vi "sys_front_panel_V1.vi"() -> ()   [LabVIEW 2024]
uses:
  <vilib>/Analysis/1siggen.llb/Ramp Pattern by Samples.vi
  <vilib>/Analysis/NI_AALBase.lvlib
panel:
  out "WRx 2 Spectrum Plot":cluster{"Y":dbl[], "Y":dbl[]}[](graph)
  in  "RTHost Selection":u16(ring) items=["192.168.1.2 C011T D83198", "192.168.1.4 C011T 50E219"]
  in  "Scan for\nConfig":bool
  out "Hardware\nBusy":bool
  in  "Toggle\nMeasurement":bool
  in  "Spectrum Sampling Period (s)":dbl caption="Measured\nOperating \nFrequency" format="%#_4f"
  out "WRx 1 Spectrum Plot":cluster{"Y":dbl[], "Y":dbl[]}[](graph)
  in  "FlexCompute Selection":u16(ring) items=["192.168.1.1 C100T 909B13", "192.168.1.3 C100T 4363DA"]
  in  "FlexSDR Selection":u16(ring) items=["192.168.1.5  S8010-01 9770BC", "192.168.1.6  S8010-01 24BD53"]
  in  "Stop Program":bool
  in  "Use Random\nDevices":bool
  in  "Scan for \nDevices":bool
  in  "?":T1(tab)
  in  "Runtime\nCalibration":bool
  in  "?":enum32{"WRx 1", "WRx 2"}(tab)
  in  "WRx 1\nGain Attenuation":i64(knob) caption="RX Gain Attenuation" min=0 max=27 step=1 scale=0.0..27.0
  in  "WRx 1\nIF Frequency":u16(ring) caption="IF Frequency" items=["1200 MHz", "1400 MHz", "3000 MHZ"]
  in  "WRx 1\nEnable Channel":bool caption="Enable \nChannel"
  in  "WRx 1\nBandwidth Mode":u16(ring) caption="Bandwidth Mode" items=["500 MHz"]
  in  "WRx 1\nGain Mode":u16(ring) caption="Gain Mode" items=["Automatic", "Fixed"]
  in  "WRx 1\nRSSI Threshold":dbl caption="RX RSSI Threshold" format="%.2f dBm"
  in  "WRx 2\nGain Mode":u16(ring) caption="Gain Mode" items=["Automatic", "Fixed"]
  in  "WRx 2\nBandwidth Mode":u16(ring) caption="Bandwidth Mode" items=["500 MHz"]
  in  "WRx 2\nEnable Channel":bool caption="Enable \nChannel"
  in  "WRx 2\nIF Frequency":u16(ring) caption="IF Frequency" items=["1200 MHz", "1400 MHz", "3000 MHZ"]
  in  "WRx 2\nGain Attenuation":i64(knob) caption="RX Gain Attenuation" min=0 max=27 step=1 scale=0.0..27.0
  in  "WRx 2\nRSSI Threshold":dbl caption="RX RSSI Threshold" format="%.2f dBm"
  in  "Update \nConfiguration":bool
  in  "Doppler\nBypass":bool
  in  "Pre-Trigger Time":dbl format="%.3f ms"
  in  "Post-Trigger Time":dbl format="%.3f ms"
  in  "Trigger Type":u16(ring) items=["GPS Time", "Anomaly Detection"]
  in  "Trigger Frequency":u16(ring) caption="Trigger Type" items=["Single", "Continuous"]
  out "WRx 2 \nGain Attenuation":dbl caption="WRx 2 Gain Attenuation" format="%.0f dBm"
  out "WRx 1 \nGain Attenuation":dbl caption="WRx 1 Gain Attenuation" format="%.0f dBm"
  in  "WRx Scan":bool
  out "WRx 1 RSSI":dbl caption="Measured\nOperating \nFrequency" format="%.2f dBm"
  in  "HW Reset":bool
  in  "Self-Cal":bool
  out "WRx 2 RSSI":dbl caption="Measured\nOperating \nFrequency" format="%.2f dBm"
  out "WRx 2 En":bool
  out "WRx 1 En":bool
  out "RTHost\nDevices":string[][](array[string])
  out "FlexCompute\nDevices":string[][](array[string])
  out "FlexSDR\nDevices":string[][](array[string])
  out "Measurement\nActive":bool
  out "GPS \nLOCK":bool
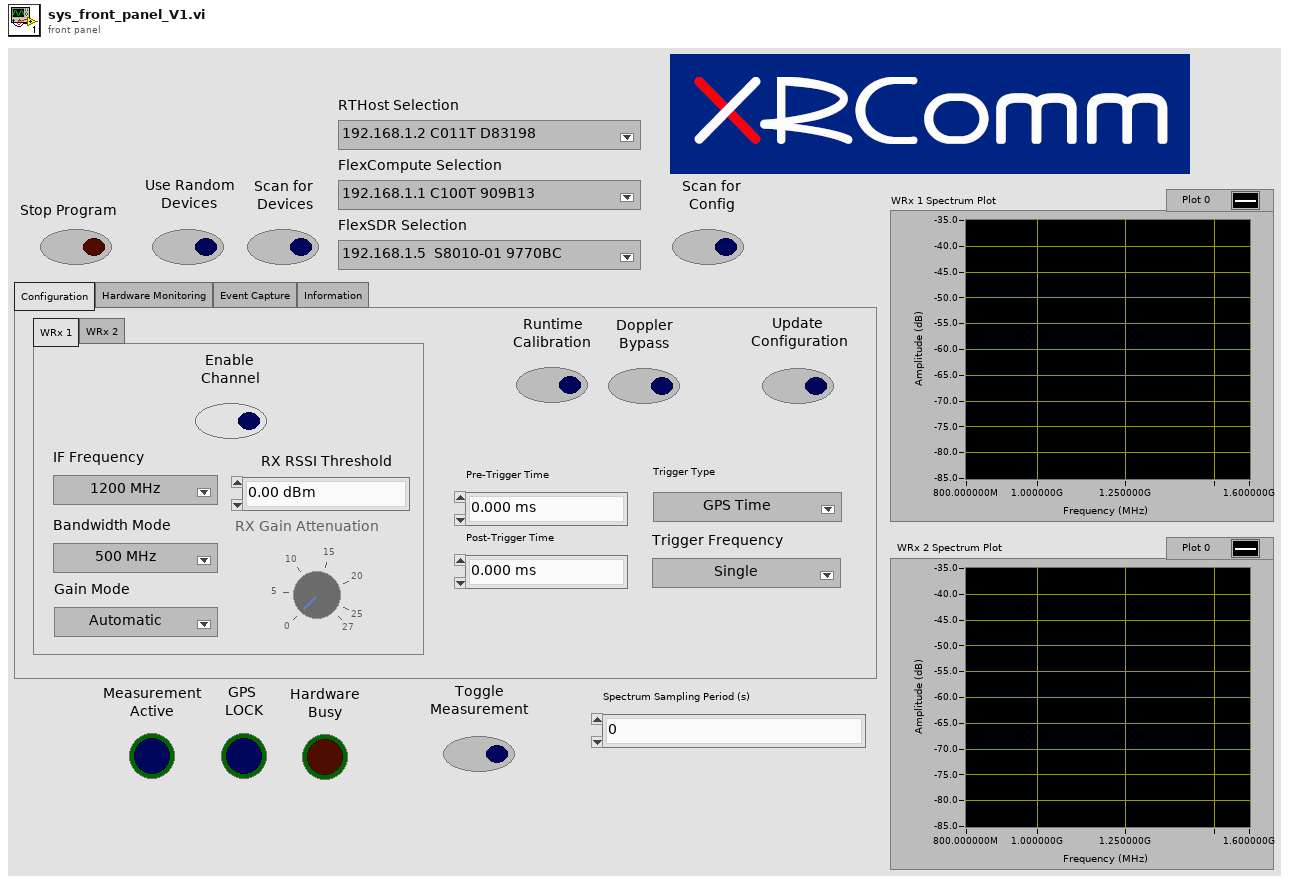
[diagram p1: front panel]
types:
  T1 = enum32{"Configuration", "Hardware Monitoring", "Event Capture", "Information"}
  T2 = enum8{"Enabled", "Disabled", "Disabled and Grayed Out"}
  T3 = cluster{"RTHost Selection":u16, "FlexCompute Selection":u16, "FlexSDR Selection":u16}
  T4 = cluster{"RTHost\nDevices":string[][], "FlexCompute\nDevices":string[][], "FlexSDR\nDevices":string[][]}
  T5 = cluster{"Doppler\nBypass":bool, "Trigger Type":u16, "Trigger Frequency":u16, "Pre-Trigger Time":dbl, "Post-Trigger Time":dbl}
  T6 = cluster{"WRx 1\nEnable Channel":bool, "WRx 1\nIF Frequency":u16, "WRx 1\nBandwidth Mode":u16, "WRx 1\nGain Mode":u16, "WRx 1\nRSSI Threshold":dbl, "WRx 1\nGain Attenuation":i64, "WRx 2\nEnable Channel":bool, "WRx 2\nIF Frequency":u16, "WRx 2\nBandwidth Mode":u16, "WRx 2\nGain Mode":u16, "WRx 2\nRSSI Threshold":dbl, "WRx 2\nGain Attenuation":i64, "Runtime\nCalibration":bool, "Measurement\nActive":bool}
  T7 = cluster{"SDR Config":cluster{"WRx 1\nEnable Channel":bool, "WRx 1\nIF Frequency":u16, "WRx 1\nBandwidth Mode":u16, "WRx 1\nGain Mode":u16, "WRx 1\nRSSI Threshold":dbl, "WRx 1\nGain Attenuation":i64, "WRx 2\nEnable Channel":bool, "WRx 2\nIF Frequency":u16, "WRx 2\nBandwidth Mode":u16, "WRx 2\nGain Mode":u16, "WRx 2\nRSSI Threshold":dbl, "WRx 2\nGain Attenuation":i64, "Runtime\nCalibration":bool, "Measurement\nActive":bool}, "Compute Config":cluster{"Doppler\nBypass":bool, "Trigger Type":u16, "Trigger Frequency":u16, "Pre-Trigger Time":dbl, "Post-Trigger Time":dbl}}
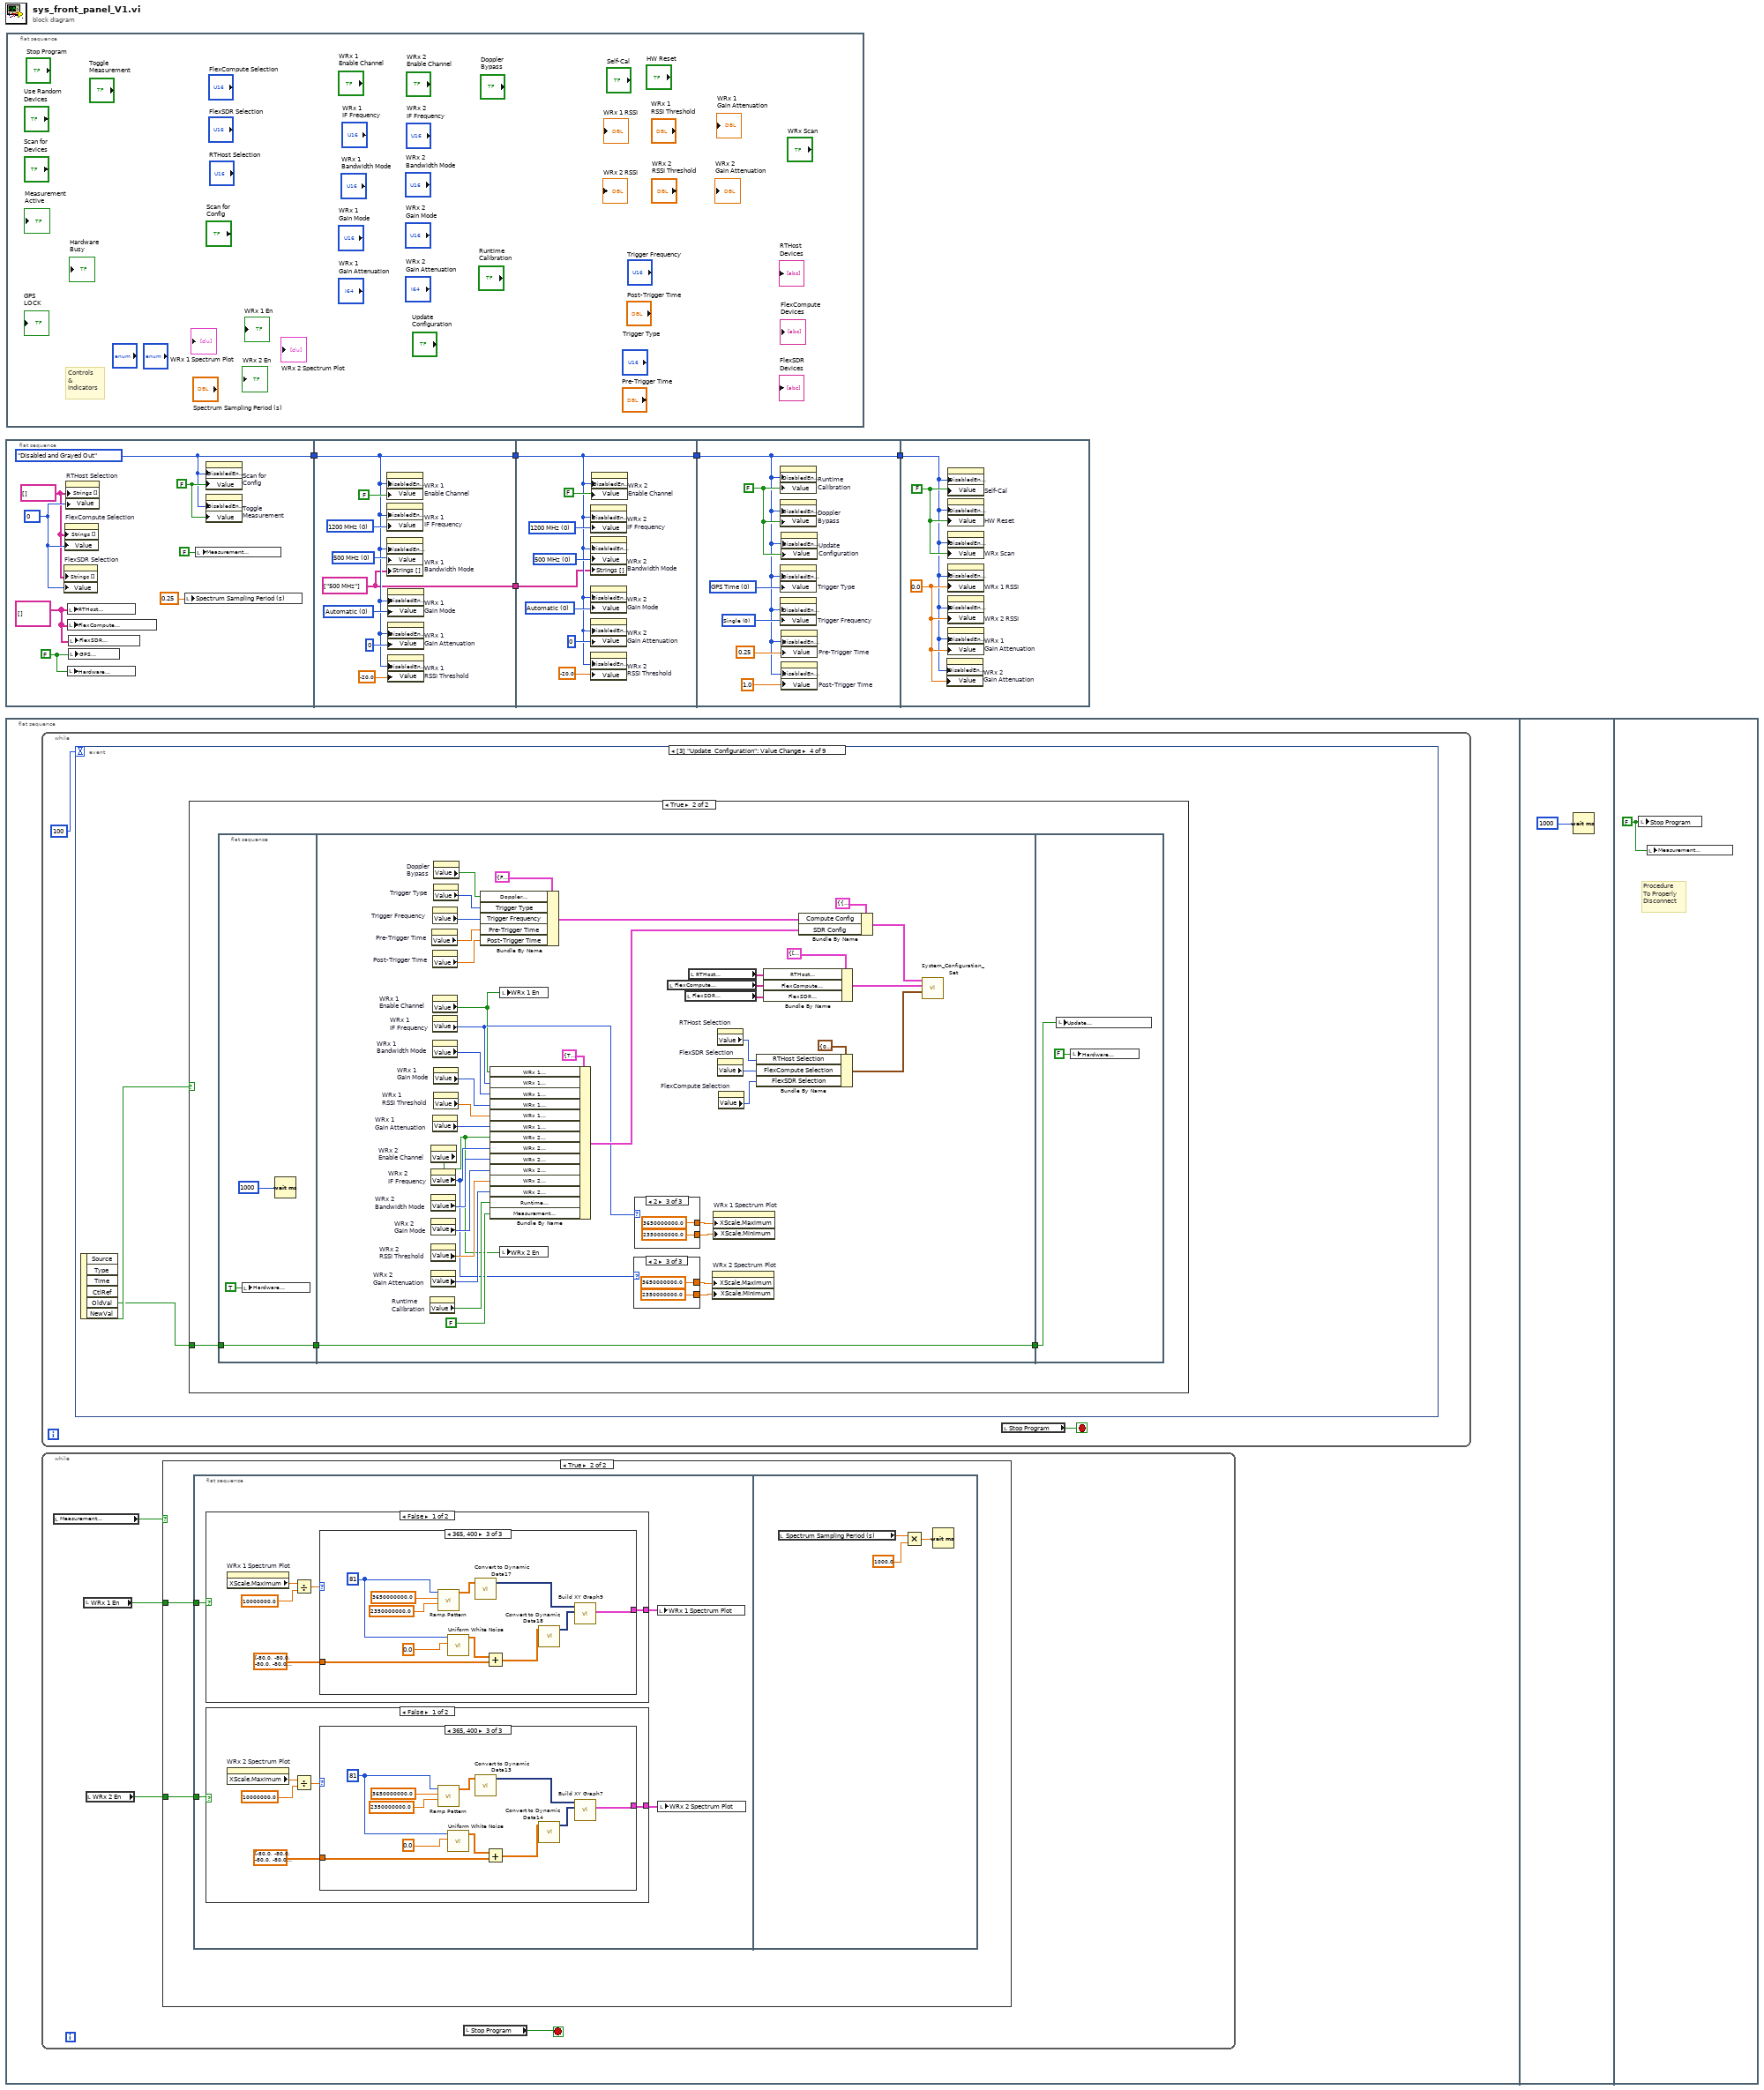
[diagram p0: block diagram]
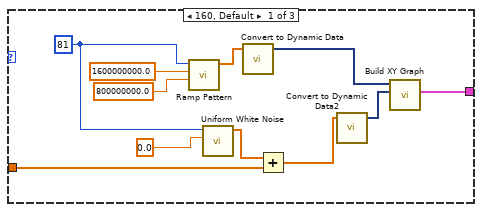
[diagram p3: hidden frame]
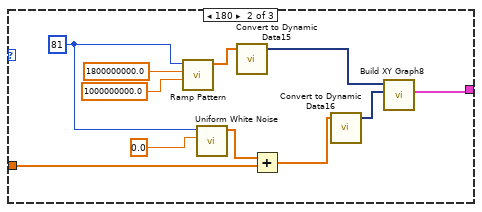
[diagram p4: hidden frame]
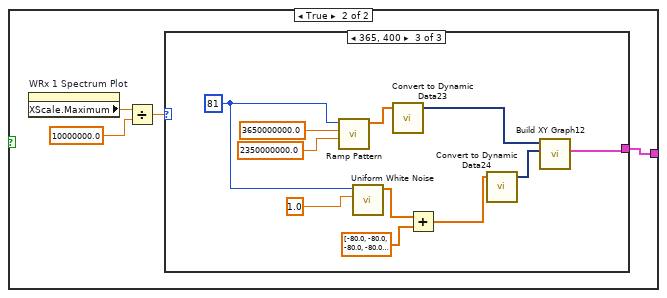
[diagram p5: hidden frame]
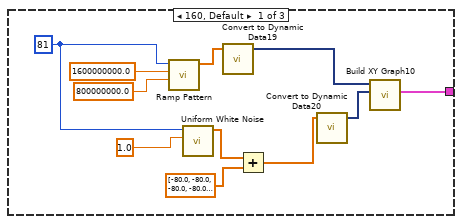
[diagram p6: hidden frame]
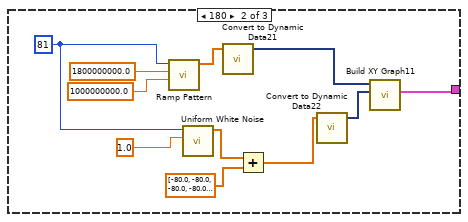
[diagram p7: hidden frame]
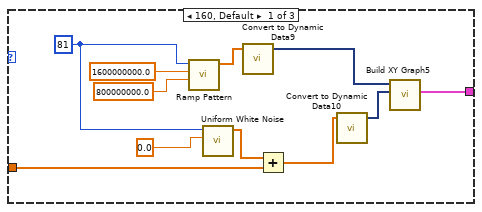
[diagram p8: hidden frame]
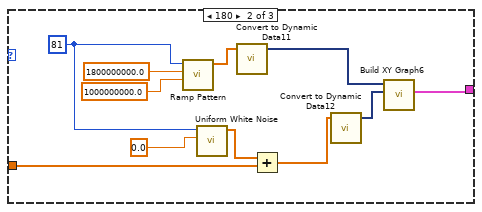
[diagram p9: hidden frame]
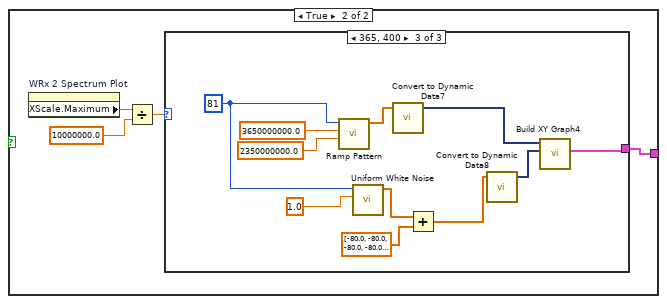
[diagram p10: hidden frame]
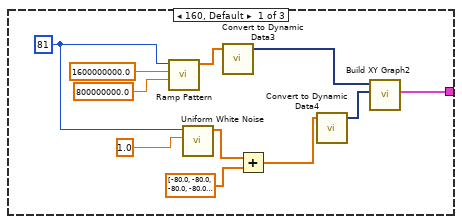
[diagram p11: hidden frame]
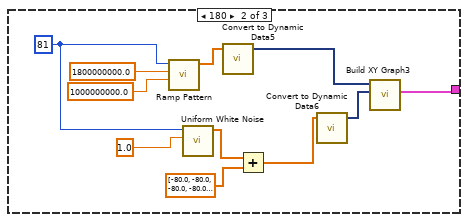
[diagram p12: hidden frame]
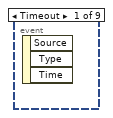
[diagram p13: hidden frame]
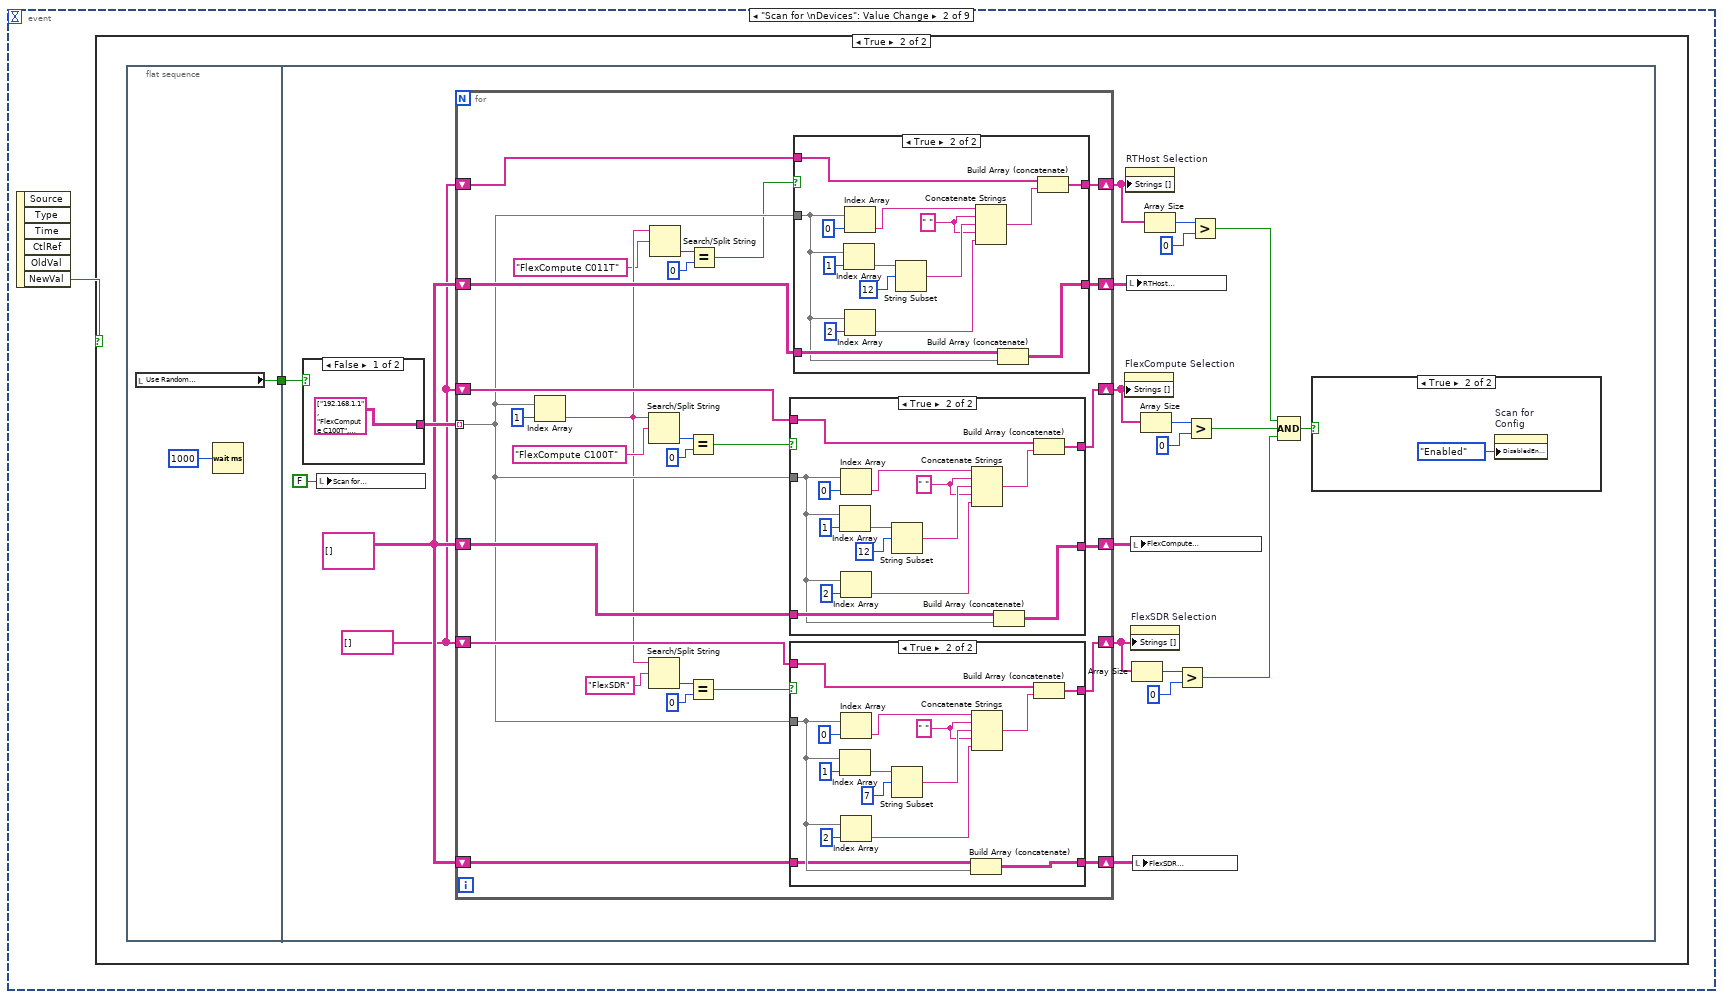
[diagram p14: hidden frame]
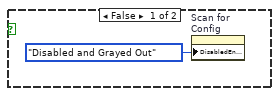
[diagram p16: hidden frame]
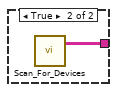
[diagram p20: hidden frame]
diagram:
  n1 = flat-sequence {
    frame #0 {
      n2 = while {
        stop <- w170 stop-if-true
        n3 = event shown="[3] \"Update  Configuration\": Value Change" {
          selector: _ -> [_ _ _ _ _ _ _ _ _]
          dyn-events: _ -> [_ _ _ _ _ _ _ _ _]
          timeout: 100 -> [_ _ _ _ _ _ _ _ _]
          event Timeout {
            n4 = event-data() -> ()  [unwired: 1 in, 3 out]
          }
          event "Scan for \nDevices": Value Change {
            n5 = event-data() -> ("NewVal"=w171:bool)  [unwired: 1 in, 5 out]
            n6 = case shown="True" w171 {
              frame False {
              }
              frame True {
                n7 = flat-sequence {
                  tunnel: [w173] -> w172
                  tunnel: w172 -> [w191]
                  frame #0 {
                    n8 = local read "Use Random\nDevices"() -> (w173:bool)
                    n9 = Wait (ms)(milliseconds to wait=u32 1000) -> ()  [unwired: 1 out]
                  }
                  frame #1 {
                    w190 = string[][] [] ("Flex Computer\nDevices 2")
                    w189 = string[] []
                    n10 = case shown="False" w191 {
                      tunnel: [string[][] [["192.168.1.1", "FlexCompute C100T", "909B13"], ["192.168.1.2", "FlexCompute C011T", "D83198"], ["192.168.1.3", "FlexCompute C100T", "4363DA"], ["192.168.1.4", "FlexCompute C011T", "50E219"], ["192.168.1.5", "FlexSDR S8010-01", "9770BC"], ["192.168.1.6", "FlexSDR S8010-01", "24BD53"]] ("Device Properties") w277] -> w194
                      frame False {
                      }
                      frame True {
                        n11 = call "Scan_For_Devices.vi"() -> ("Device Properties"=w277:string[][])  [unwired: 3 in]
                      }
                    }
                    n12 = local write "Scan for \nDevices"(FALSE ("Scan for \nDevices")) -> ()
                    n13 = for {
                      tunnel: w194 -> [w201] mode=indexing
                      shift-right: [w219] -> w182
                      shift-left: w189 -> [w220]
                      shift-right: [w218] -> w179
                      shift-left: w189 -> [w213]
                      shift-right: [w211] -> w193
                      shift-left: w190 -> [w212]
                      shift-right: [w209] -> w192
                      shift-left: w190 -> [w210]
                      shift-right: [w206] -> w188
                      shift-left: w190 -> [w207]
                      shift-right: [w205] -> w187
                      shift-left: w189 -> [w204]
                      n14 = Index Array(array=w201, index=1) -> (element=w200:string)
                      n15 = Search/Split String(string=w200, search string/char (-)="FlexCompute C100T") -> (offset of match=w223:i32)  [unwired: 1 in, 2 out]
                      n16 = Search/Split String(string=w200, search string/char (-)="FlexSDR") -> (offset of match=w217:i32)  [unwired: 1 in, 2 out]
                      n17 = Search/Split String(string=w200, search string/char (-)="FlexCompute C011T") -> (offset of match=w203:i32)  [unwired: 1 in, 2 out]
                      n18 = Equal?(x=w223, y=0) -> (x = y?=w221:bool)
                      n19 = Equal?(x=w217, y=0) -> (x = y?=w214:bool)
                      n20 = Equal?(x=w203, y=0) -> (x = y?=w198:bool)
                      n21 = case shown="True" w221 {
                        tunnel: w201 -> [_ w262]
                        tunnel: w220 -> [w260 w265]
                        tunnel: [w260 w264] -> w219
                        tunnel: w212 -> [w259 w263]
                        tunnel: [w259 w261] -> w211
                        frame False {
                        }
                        frame True {
                          w268 = " " ("string")
                          n22 = Index Array(array=w262, index=1) -> (element=w272:string)
                          n23 = Index Array(array=w262, index=0) -> (element=w270:string)
                          n24 = Index Array(array=w262, index=2) -> (element=w267:string)
                          n25 = String Subset(string=w272, offset (0)=12) -> (substring=w269:string)  [unwired: 1 in]
                          n26 = Concatenate Strings(w270, w268, w269, w268, w267) -> (w266:string)
                          n27 = Build Array (concatenate)(w263, w262) -> (w261:string[][])
                          n28 = Build Array (concatenate)(w265, w266) -> (w264:string[])
                        }
                      }
                      n29 = case shown="True" w214 {
                        tunnel: w201 -> [_ w246]
                        tunnel: w213 -> [w243 w248]
                        tunnel: [w243 w247] -> w218
                        tunnel: w210 -> [w242 w245]
                        tunnel: [w242 w244] -> w209
                        frame False {
                        }
                        frame True {
                          w251 = " " ("string")
                          n30 = Index Array(array=w246, index=1) -> (element=w255:string)
                          n31 = Index Array(array=w246, index=0) -> (element=w253:string)
                          n32 = Index Array(array=w246, index=2) -> (element=w250:string)
                          n33 = String Subset(string=w255, offset (0)=7) -> (substring=w252:string)  [unwired: 1 in]
                          n34 = Build Array (concatenate)(w245, w246) -> (w244:string[][])
                          n35 = Concatenate Strings(w253, w251, w252, w251, w250) -> (w249:string)
                          n36 = Build Array (concatenate)(w248, w249) -> (w247:string[])
                        }
                      }
                      n37 = case shown="True" w198 {
                        tunnel: w201 -> [_ w228]
                        tunnel: w204 -> [w226 w231]
                        tunnel: [w226 w230] -> w205
                        tunnel: w207 -> [w225 w229]
                        tunnel: [w225 w227] -> w206
                        frame False {
                        }
                        frame True {
                          w234 = " " ("string")
                          n38 = Index Array(array=w228, index=1) -> (element=w238:string)
                          n39 = Index Array(array=w228, index=0) -> (element=w236:string)
                          n40 = Index Array(array=w228, index=2) -> (element=w233:string)
                          n41 = String Subset(string=w238, offset (0)=12) -> (substring=w235:string)  [unwired: 1 in]
                          n42 = Concatenate Strings(w236, w234, w235, w234, w233) -> (w232:string)
                          n43 = Build Array (concatenate)(w229, w228) -> (w227:string[][])
                          n44 = Build Array (concatenate)(w231, w232) -> (w230:string[])
                        }
                      }
                    }
                    n45 = property on="FlexCompute Selection" class="Ring (strict)"("Strings []"=w182) -> ()  [unwired: 2 in, 2 out]
                    n46 = property on="RTHost Selection" class="Ring (strict)"("Strings []"=w187) -> ()  [unwired: 2 in, 2 out]
                    n47 = local write "RTHost\nDevices"(w188) -> ()
                    n48 = local write "FlexCompute\nDevices"(w193) -> ()
                    n49 = property on="FlexSDR Selection" class="Ring (strict)"("Strings []"=w179) -> ()  [unwired: 2 in, 2 out]
                    n50 = Array Size(array=w179) -> (size(s)=w181:i32)
                    n51 = local write "FlexSDR\nDevices"(w192) -> ()
                    n52 = Array Size(array=w182) -> (size(s)=w184:i32)
                    n53 = Array Size(array=w187) -> (size(s)=w186:i32)
                    n54 = Greater?(x=w181, y=0) -> (0:w176:bool)
                    n55 = Greater?(x=w184, y=0) -> (0:w177:bool)
                    n56 = Greater?(x=w186, y=0) -> (0:w178:bool)
                    n57 = Compound Arithmetic op=AND(w178, w177, w176) -> (w175:bool)
                    n58 = case shown="True" w175 {
                      frame False {
                        n59 = property on="Scan for\nConfig" class="Bool (strict)"("DisabledEnum"=T2."Disabled and Grayed Out" ("Disabled")) -> ()  [unwired: 2 in, 2 out]
                      }
                      frame True {
                        n60 = property on="Scan for\nConfig" class="Bool (strict)"("DisabledEnum"=T2."Enabled" ("Disabled")) -> ()  [unwired: 2 in, 2 out]
                      }
                    }
                  }
                }
              }
            }
          }
          event "Scan for\nConfig": Value Change {
            n61 = event-data() -> ("NewVal"=w279:bool)  [unwired: 1 in, 5 out]
            n62 = flat-sequence {
              tunnel: w279 -> [w281]
              tunnel: [w281] -> w278
              tunnel: w278 -> [w282]
              frame #0 {
                n63 = Wait (ms)(milliseconds to wait=u32 1000) -> ()  [unwired: 1 out]
              }
              frame #1 {
                n64 = case shown="True" w282 {
                  frame False {
                  }
                  frame True {
                    w308 = 0.0 ("WRx 1 RSSI")
                    w297 = FALSE ("HW Reset")
                    w298 = T2."Enabled" ("Disabled")
                    n65 = local read "FlexCompute\nDevices"() -> (w322:string[][])
                    n66 = local read "FlexSDR\nDevices"() -> (w321:string[][])
                    n67 = local read "RTHost\nDevices"() -> (w323:string[][])
                    n68 = property on="FlexCompute Selection" class="Ring (strict)"() -> ("Value"=w325:u16)  [unwired: 2 in, 2 out]
                    n69 = property on="FlexSDR Selection" class="Ring (strict)"() -> ("Value"=w324:u16)  [unwired: 2 in, 2 out]
                    n70 = property on="RTHost Selection" class="Ring (strict)"() -> ("Value"=w327:u16)  [unwired: 2 in, 2 out]
                    n71 = property on="WRx 2 \nGain Attenuation" class="DigNum (strict)"("DisabledEnum"=w298, "Value"=w308) -> ()  [unwired: 2 in, 2 out]
                    n72 = property on="Self-Cal" class="Bool (strict)"("DisabledEnum"=w298, "Value"=w297) -> ()  [unwired: 2 in, 2 out]
                    n73 = property on="HW Reset" class="Bool (strict)"("DisabledEnum"=w298, "Value"=w297) -> ()  [unwired: 2 in, 2 out]
                    n74 = property on="WRx Scan" class="Bool (strict)"("DisabledEnum"=w298, "Value"=w297) -> ()  [unwired: 2 in, 2 out]
                    n75 = property on="WRx 1 RSSI" class="DigNum (strict)"("DisabledEnum"=w298, "Value"=w308) -> ()  [unwired: 2 in, 2 out]
                    n76 = property on="WRx 2 RSSI" class="DigNum (strict)"("DisabledEnum"=w298, "Value"=w308) -> ()  [unwired: 2 in, 2 out]
                    n77 = property on="WRx 1 \nGain Attenuation" class="DigNum (strict)"("DisabledEnum"=w298, "Value"=w308) -> ()  [unwired: 2 in, 2 out]
                    n78 = property on="Toggle\nMeasurement" class="Bool (strict)"("DisabledEnum"=w298, "Value"=w297) -> ()  [unwired: 2 in, 2 out]
                    n79 = Bundle By Name(cluster=T3 {"RTHost Selection"=0, "FlexCompute Selection"=0, "FlexSDR Selection"=0} ("Device Selection 2"), "RTHost Selection"=w327, "FlexCompute Selection"=w325, "FlexSDR Selection"=w324) -> (w296:T3)
                    n80 = Bundle By Name(cluster=T4 {"RTHost\nDevices"=[], "FlexCompute\nDevices"=[], "FlexSDR\nDevices"=[]} ("Devices 2"), "RTHost\nDevices"=w323, "FlexCompute\nDevices"=w322, "FlexSDR\nDevices"=w321) -> (w295:T4)
                    n81 = call "System_Configuration_Get.vi"("Device Selection"=w296, "Devices"=w295) -> ("Config"=w320:T7)  [unwired: 3 in, 1 out]
                    n82 = Unbundle By Name(w320) -> ("Compute Config"=w319:T5, "SDR Config"=w307:T6)
                    n83 = Unbundle By Name(w307) -> ("WRx 1\nEnable Channel"=w290:bool, "WRx 1\nIF Frequency"=w315:u16, "WRx 1\nBandwidth Mode"=w318:u16, "WRx 1\nGain Mode"=w287:u16, "WRx 1\nRSSI Threshold"=w316:dbl, "WRx 1\nGain Attenuation"=w317:i64)
                    n84 = case shown="1" w287 {
                      tunnel: [T2."Disabled and Grayed Out" ("Disabled") T2."Enabled" ("Disabled")] -> w288
                      tunnel: [T2."Enabled" ("Disabled") T2."Disabled and Grayed Out" ("Disabled")] -> w286
                      frame 0, Default {
                      }
                      frame 1 {
                      }
                    }
                    n85 = case shown="0, Default" w315 {
                      tunnel: [string[] ["500 MHz"] ("Strings []") string[] ["500 MHz"] ("Strings []") string[] ["500 MHz", "1000 MHz"] ("Strings []")] -> w314
                      tunnel: [1600000000.0 ("X Scale.Range:Maximum") 1800000000.0 ("X Scale.Range:Maximum") 3650000000.0 ("X Scale.Range:Maximum")] -> w294
                      tunnel: [800000000.0 ("X Scale.Range:Minimum") 1000000000.0 ("X Scale.Range:Minimum") 2350000000.0 ("X Scale.Range:Minimum")] -> w293
                      frame 0, Default {
                      }
                      frame 1 {
                      }
                      frame 2 {
                      }
                    }
                    n86 = local write "WRx 1 En"(w290) -> ()
                    n87 = property on="WRx 1\nEnable Channel" class="Bool (strict)"("DisabledEnum"=w298, "Value"=w290) -> ()  [unwired: 2 in, 2 out]
                    n88 = property on="WRx 1\nIF Frequency" class="Ring (strict)"("DisabledEnum"=w298, "Value"=w315) -> ()  [unwired: 2 in, 2 out]
                    n89 = property on="WRx 1\nBandwidth Mode" class="Ring (strict)"("DisabledEnum"=w298, "Value"=w318, "Strings []"=w314) -> ()  [unwired: 2 in, 2 out]
                    n90 = property on="WRx 1\nGain Mode" class="Ring (strict)"("DisabledEnum"=w298, "Value"=w287) -> ()  [unwired: 2 in, 2 out]
                    n91 = property on="WRx 1\nGain Attenuation" class="Knob (strict)"("DisabledEnum"=w288, "Value"=w317) -> ()  [unwired: 2 in, 2 out]
                    n92 = property on="WRx 1\nRSSI Threshold" class="DigNum (strict)"("DisabledEnum"=w286, "Value"=w316) -> ()  [unwired: 2 in, 2 out]
                    n93 = property on="WRx 1 Spectrum Plot" class="XYGraph (strict)"("XScale.Maximum"=w294, "XScale.Minimum"=w293) -> ()  [unwired: 2 in, 2 out]
                    n94 = Unbundle By Name(w307) -> ("Measurement\nActive"=w299:bool, "Runtime\nCalibration"=w300:bool, "WRx 2\nEnable Channel"=w289:bool, "WRx 2\nIF Frequency"=w310:u16, "WRx 2\nBandwidth Mode"=w313:u16, "WRx 2\nGain Mode"=w283:u16, "WRx 2\nRSSI Threshold"=w312:dbl, "WRx 2\nGain Attenuation"=w311:i64)  [unwired: 1 out]
                    n95 = case shown="1" w283 {
                      tunnel: [T2."Disabled and Grayed Out" ("Disabled") T2."Enabled" ("Disabled")] -> w285
                      tunnel: [T2."Enabled" ("Disabled") T2."Disabled and Grayed Out" ("Disabled")] -> w284
                      frame 0, Default {
                      }
                      frame 1 {
                      }
                    }
                    n96 = local write "Measurement\nActive"(w299) -> ()
                    n97 = case shown="0, Default" w310 {
                      tunnel: [string[] ["500 MHz"] ("Strings []") string[] ["500 MHz"] ("Strings []") string[] ["500 MHz", "1000 MHz"] ("Strings []")] -> w309
                      tunnel: [1600000000.0 ("X Scale.Range:Maximum") 1800000000.0 ("X Scale.Range:Maximum") 3650000000.0 ("X Scale.Range:Maximum")] -> w292
                      tunnel: [800000000.0 ("X Scale.Range:Minimum") 1000000000.0 ("X Scale.Range:Minimum") 2350000000.0 ("X Scale.Range:Minimum")] -> w291
                      frame 0, Default {
                      }
                      frame 1 {
                      }
                      frame 2 {
                      }
                    }
                    n98 = Unbundle By Name(w319) -> ("Doppler\nBypass"=w302:bool, "Trigger Type"=w303:u16, "Trigger Frequency"=w304:u16, "Pre-Trigger Time"=w305:dbl, "Post-Trigger Time"=w306:dbl)
                    n99 = local write "WRx 2 En"(w289) -> ()
                    n100 = property on="WRx 2\nIF Frequency" class="Ring (strict)"("DisabledEnum"=w298, "Value"=w310) -> ()  [unwired: 2 in, 2 out]
                    n101 = property on="WRx 2\nBandwidth Mode" class="Ring (strict)"("DisabledEnum"=w298, "Value"=w313, "Strings []"=w309) -> ()  [unwired: 2 in, 2 out]
                    n102 = property on="WRx 2\nGain Mode" class="Ring (strict)"("DisabledEnum"=w298, "Value"=w283) -> ()  [unwired: 2 in, 2 out]
                    n103 = property on="WRx 2\nGain Attenuation" class="Knob (strict)"("DisabledEnum"=w285, "Value"=w311) -> ()  [unwired: 2 in, 2 out]
                    n104 = property on="WRx 2\nRSSI Threshold" class="DigNum (strict)"("DisabledEnum"=w284, "Value"=w312) -> ()  [unwired: 2 in, 2 out]
                    n105 = property on="WRx 2\nEnable Channel" class="Bool (strict)"("DisabledEnum"=w298, "Value"=w289) -> ()  [unwired: 2 in, 2 out]
                    n106 = property on="WRx 2 Spectrum Plot" class="XYGraph (strict)"("XScale.Maximum"=w292, "XScale.Minimum"=w291) -> ()  [unwired: 2 in, 2 out]
                    n107 = property on="Runtime\nCalibration" class="Bool (strict)"("DisabledEnum"=w298, "Value"=w300) -> ()  [unwired: 2 in, 2 out]
                    n108 = property on="Doppler\nBypass" class="Bool (strict)"("DisabledEnum"=w298, "Value"=w302) -> ()  [unwired: 2 in, 2 out]
                    n109 = property on="Trigger Type" class="Ring (strict)"("DisabledEnum"=w298, "Value"=w303) -> ()  [unwired: 2 in, 2 out]
                    n110 = property on="Trigger Frequency" class="Ring (strict)"("DisabledEnum"=w298, "Value"=w304) -> ()  [unwired: 2 in, 2 out]
                    n111 = property on="Update \nConfiguration" class="Bool (strict)"("DisabledEnum"=w298, "Value"=FALSE ("Update \nConfiguration")) -> ()  [unwired: 2 in, 2 out]
                    n112 = property on="Pre-Trigger Time" class="DigNum (strict)"("DisabledEnum"=w298, "Value"=w305) -> ()  [unwired: 2 in, 2 out]
                    n113 = property on="Post-Trigger Time" class="DigNum (strict)"("DisabledEnum"=w298, "Value"=w306) -> ()  [unwired: 2 in, 2 out]
                  }
                }
              }
              frame #2 {
                n114 = local write "Scan for\nConfig"(FALSE ("Scan for\nConfig")) -> ()
              }
            }
          }
          event "Update \nConfiguration": Value Change {
            n115 = event-data() -> ("OldVal"=w356:bool, "NewVal"=w357:bool)  [unwired: 1 in, 4 out]
            n116 = case shown="True" w357 {
              tunnel: w356 -> [_ w359]
              frame False {
              }
              frame True {
                n117 = flat-sequence {
                  tunnel: [w362] -> w360
                  tunnel: w359 -> [w362]
                  tunnel: w360 -> [w364]
                  tunnel: [w364] -> w358
                  tunnel: w358 -> [w416]
                  frame #0 {
                    n118 = local write "Hardware\nBusy"(TRUE ("Hardware\nBusy")) -> ()
                    n119 = Wait (ms)(milliseconds to wait=u32 1000) -> ()  [unwired: 1 out]
                  }
                  frame #1 {
                    n120 = property on="Runtime\nCalibration" class="Bool (strict)"() -> ("Value"=w396:bool)  [unwired: 2 in, 2 out]
                    n121 = property on="WRx 2\nIF Frequency" class="Ring (strict)"() -> ("Value"=w367:u16)  [unwired: 2 in, 2 out]
                    n122 = property on="WRx 2\nBandwidth Mode" class="Ring (strict)"() -> ("Value"=w391:u16)  [unwired: 2 in, 2 out]
                    n123 = property on="WRx 2\nGain Mode" class="Ring (strict)"() -> ("Value"=w392:u16)  [unwired: 2 in, 2 out]
                    n124 = property on="WRx 2\nRSSI Threshold" class="DigNum (strict)"() -> ("Value"=w393:dbl)  [unwired: 2 in, 2 out]
                    n125 = property on="WRx 2\nGain Attenuation" class="Knob (strict)"() -> ("Value"=w394:i64)  [unwired: 2 in, 2 out]
                    n126 = property on="WRx 2\nEnable Channel" class="Bool (strict)"() -> ("Value"=w366:bool)  [unwired: 2 in, 2 out]
                    n127 = property on="Pre-Trigger Time" class="DigNum (strict)"() -> ("Value"=w386:dbl)  [unwired: 2 in, 2 out]
                    n128 = property on="Trigger Frequency" class="Ring (strict)"() -> ("Value"=w390:u16)  [unwired: 2 in, 2 out]
                    n129 = property on="Post-Trigger Time" class="DigNum (strict)"() -> ("Value"=w387:dbl)  [unwired: 2 in, 2 out]
                    n130 = property on="WRx 1\nEnable Channel" class="Bool (strict)"() -> ("Value"=w365:bool)  [unwired: 2 in, 2 out]
                    n131 = property on="WRx 1\nIF Frequency" class="Ring (strict)"() -> ("Value"=w370:u16)  [unwired: 2 in, 2 out]
                    n132 = property on="WRx 1\nBandwidth Mode" class="Ring (strict)"() -> ("Value"=w400:u16)  [unwired: 2 in, 2 out]
                    n133 = property on="WRx 1\nGain Attenuation" class="Knob (strict)"() -> ("Value"=w397:i64)  [unwired: 2 in, 2 out]
                    n134 = property on="Trigger Type" class="Ring (strict)"() -> ("Value"=w388:u16)  [unwired: 2 in, 2 out]
                    n135 = property on="WRx 1\nGain Mode" class="Ring (strict)"() -> ("Value"=w399:u16)  [unwired: 2 in, 2 out]
                    n136 = property on="WRx 1\nRSSI Threshold" class="DigNum (strict)"() -> ("Value"=w398:dbl)  [unwired: 2 in, 2 out]
                    n137 = property on="Doppler\nBypass" class="Bool (strict)"() -> ("Value"=w389:bool)  [unwired: 2 in, 2 out]
                    n138 = Bundle By Name(cluster=T5 {"Doppler\nBypass"=FALSE, "Trigger Type"=0, "Trigger Frequency"=0, "Pre-Trigger Time"=0.25, "Post-Trigger Time"=1.0} ("Compute Config"), "Doppler\nBypass"=w389, "Trigger Type"=w388, "Trigger Frequency"=w390, "Pre-Trigger Time"=w386, "Post-Trigger Time"=w387) -> (w384:T5)
                    n139 = Bundle By Name(cluster=T6 {"WRx 1\nEnable Channel"=TRUE, "WRx 1\nIF Frequency"=2, "WRx 1\nBandwidth Mode"=0, "WRx 1\nGain Mode"=0, "WRx 1\nRSSI Threshold"=-20.0, "WRx 1\nGain Attenuation"=0, "WRx 2\nEnable Channel"=FALSE, "WRx 2\nIF Frequency"=0, "WRx 2\nBandwidth Mode"=0, "WRx 2\nGain Mode"=0, "WRx 2\nRSSI Threshold"=-20.0, "WRx 2\nGain Attenuation"=0, "Runtime\nCalibration"=FALSE, "Measurement\nActive"=FALSE} ("SDR Config"), "WRx 1\nEnable Channel"=w365, "WRx 1\nIF Frequency"=w370, "WRx 1\nBandwidth Mode"=w400, "WRx 1\nGain Mode"=w399, "WRx 1\nRSSI Threshold"=w398, "WRx 1\nGain Attenuation"=w397, "WRx 2\nEnable Channel"=w366, "WRx 2\nIF Frequency"=w367, "WRx 2\nBandwidth Mode"=w391, "WRx 2\nGain Mode"=w392, "WRx 2\nRSSI Threshold"=w393, "WRx 2\nGain Attenuation"=w394, "Runtime\nCalibration"=w396, "Measurement\nActive"=FALSE ("Measurement\nActive")) -> (w385:T6)
                    n140 = local write "WRx 1 En"(w365) -> ()
                    n141 = local write "WRx 2 En"(w366) -> ()
                    n142 = case shown="2" w367 {
                      tunnel: [1600000000.0 ("X Scale.Range:Maximum") 1800000000.0 ("X Scale.Range:Maximum") 3650000000.0 ("X Scale.Range:Maximum")] -> w369
                      tunnel: [800000000.0 ("X Scale.Range:Minimum") 1000000000.0 ("X Scale.Range:Minimum") 2350000000.0 ("X Scale.Range:Minimum")] -> w368
                      frame 0, Default {
                      }
                      frame 1 {
                      }
                      frame 2 {
                      }
                    }
                    n143 = case shown="2" w370 {
                      tunnel: [1600000000.0 ("X Scale.Range:Maximum") 1800000000.0 ("X Scale.Range:Maximum") 3650000000.0 ("X Scale.Range:Maximum")] -> w372
                      tunnel: [800000000.0 ("X Scale.Range:Minimum") 1000000000.0 ("X Scale.Range:Minimum") 2350000000.0 ("X Scale.Range:Minimum")] -> w371
                      frame 0, Default {
                      }
                      frame 1 {
                      }
                      frame 2 {
                      }
                    }
                    n144 = local read "FlexCompute\nDevices"() -> (w381:string[][])
                    n145 = local read "FlexSDR\nDevices"() -> (w379:string[][])
                    n146 = local read "RTHost\nDevices"() -> (w380:string[][])
                    n147 = property on="WRx 2 Spectrum Plot" class="XYGraph (strict)"("XScale.Maximum"=w369, "XScale.Minimum"=w368) -> ()  [unwired: 2 in, 2 out]
                    n148 = property on="WRx 1 Spectrum Plot" class="XYGraph (strict)"("XScale.Maximum"=w372, "XScale.Minimum"=w371) -> ()  [unwired: 2 in, 2 out]
                    n149 = property on="RTHost Selection" class="Ring (strict)"() -> ("Value"=w376:u16)  [unwired: 2 in, 2 out]
                    n150 = property on="FlexSDR Selection" class="Ring (strict)"() -> ("Value"=w375:u16)  [unwired: 2 in, 2 out]
                    n151 = property on="FlexCompute Selection" class="Ring (strict)"() -> ("Value"=w374:u16)  [unwired: 2 in, 2 out]
                    n152 = Bundle By Name(cluster=T3 {"RTHost Selection"=0, "FlexCompute Selection"=0, "FlexSDR Selection"=0} ("Device Selection"), "RTHost Selection"=w376, "FlexCompute Selection"=w375, "FlexSDR Selection"=w374) -> (w373:T3)
                    n153 = Bundle By Name(cluster=T4 {"RTHost\nDevices"=[["192.168.1.2", "FlexCompute C011T", "D83198"], ["192.168.1.4", "FlexCompute C011T", "50E219"]], "FlexCompute\nDevices"=[["192.168.1.1", "FlexCompute C100T", "909B13"], ["192.168.1.3", "FlexCompute C100T", "4363DA"]], "FlexSDR\nDevices"=[["192.168.1.5", "FlexSDR S8010-01", "9770BC"], ["192.168.1.6", "FlexSDR S8010-01", "24BD53"]]} ("Devices"), "RTHost\nDevices"=w380, "FlexCompute\nDevices"=w381, "FlexSDR\nDevices"=w379) -> (w378:T4)
                    n154 = Bundle By Name(cluster=T7 {"SDR Config"={"WRx 1\nEnable Channel"=TRUE, "WRx 1\nIF Frequency"=2, "WRx 1\nBandwidth Mode"=0, "WRx 1\nGain Mode"=0, "WRx 1\nRSSI Threshold"=-20.0, "WRx 1\nGain Attenuation"=0, "WRx 2\nEnable Channel"=FALSE, "WRx 2\nIF Frequency"=0, "WRx 2\nBandwidth Mode"=0, "WRx 2\nGain Mode"=0, "WRx 2\nRSSI Threshold"=-20.0, "WRx 2\nGain Attenuation"=0, "Runtime\nCalibration"=FALSE, "Measurement\nActive"=FALSE}, "Compute Config"={"Doppler\nBypass"=FALSE, "Trigger Type"=0, "Trigger Frequency"=0, "Pre-Trigger Time"=0.25, "Post-Trigger Time"=1.0}} ("Config"), "Compute Config"=w384, "SDR Config"=w385) -> (w383:T7)
                    n155 = call "System_Configuration_Set.vi"("Device Selection"=w373, "Devices"=w378, "Config"=w383) -> ()  [unwired: 4 in]
                  }
                  frame #2 {
                    n156 = local write "Update \nConfiguration"(w416) -> ()
                    n157 = local write "Hardware\nBusy"(FALSE ("Hardware\nBusy")) -> ()
                  }
                }
              }
            }
          }
          event "WRx 1\nIF Frequency": Value Change {
            n158 = event-data() -> ("NewVal"=w418:u16)  [unwired: 1 in, 5 out]
            n159 = case shown="0, 1, Default" w418 {
              frame 0, 1, Default {
                w419 = u16 0 items=["500 MHz"] ("WRx 1\nBandwidth Mode")
                n160 = property on="WRx 1\nBandwidth Mode" class="Ring (strict)"("Strings []"=string[] ["500 MHz"], "Value"=w419) -> ()  [unwired: 2 in, 2 out]
              }
              frame 2 {
                w421 = u16 1 items=["500 MHz", "1000 MHz"] ("WRx 1\nBandwidth Mode")
                n161 = property on="WRx 1\nBandwidth Mode" class="Ring (strict)"("Strings []"=string[] ["500 MHz", "1000 MHz"], "Value"=w421) -> ()  [unwired: 2 in, 2 out]
              }
            }
          }
          event "WRx 2\nIF Frequency": Value Change {
            n162 = event-data() -> ("NewVal"=w423:u16)  [unwired: 1 in, 5 out]
            n163 = case shown="0, 1, Default" w423 {
              frame 0, 1, Default {
                w424 = u16 0 items=["500 MHz"] ("WRx 1\nBandwidth Mode")
                n164 = property on="WRx 2\nBandwidth Mode" class="Ring (strict)"("Strings []"=string[] ["500 MHz"], "Value"=w424) -> ()  [unwired: 2 in, 2 out]
              }
              frame 2 {
                w426 = u16 1 items=["500 MHz", "1000 MHz"] ("WRx 1\nBandwidth Mode")
                n165 = property on="WRx 2\nBandwidth Mode" class="Ring (strict)"("Strings []"=string[] ["500 MHz", "1000 MHz"], "Value"=w426) -> ()  [unwired: 2 in, 2 out]
              }
            }
          }
          event "WRx 1\nGain Mode": Value Change {
            n166 = event-data() -> ("NewVal"=w432:u16)  [unwired: 1 in, 5 out]
            n167 = case shown="0, Default" w432 {
              tunnel: [T2."Disabled and Grayed Out" ("Disabled") T2."Enabled" ("Disabled")] -> w430
              tunnel: [T2."Enabled" ("Disabled") T2."Disabled and Grayed Out" ("Disabled")] -> w428
              frame 0, Default {
              }
              frame 1 {
              }
            }
            n168 = property on="WRx 1\nRSSI Threshold" class="DigNum (strict)"("DisabledEnum"=w428, "Value"=-20.0 ("WRx 1\nRSSI Threshold")) -> ()  [unwired: 2 in, 2 out]
            n169 = property on="WRx 1\nGain Attenuation" class="Knob (strict)"("DisabledEnum"=w430, "Value"=i64 0 ("WRx 1\nGain Attenuation")) -> ()  [unwired: 2 in, 2 out]
          }
          event "WRx 2\nGain Mode": Value Change {
            n170 = event-data() -> ("NewVal"=w441:u16)  [unwired: 1 in, 5 out]
            n171 = case shown="0, Default" w441 {
              tunnel: [T2."Disabled and Grayed Out" ("Disabled") T2."Enabled" ("Disabled")] -> w440
              tunnel: [T2."Enabled" ("Disabled") T2."Disabled and Grayed Out" ("Disabled")] -> w437
              frame 0, Default {
              }
              frame 1 {
              }
            }
            n172 = property on="WRx 2\nGain Attenuation" class="Knob (strict)"("DisabledEnum"=w440, "Value"=i64 0 ("WRx 1\nGain Attenuation")) -> ()  [unwired: 2 in, 2 out]
            n173 = property on="WRx 2\nRSSI Threshold" class="DigNum (strict)"("DisabledEnum"=w437, "Value"=-20.0 ("WRx 1\nRSSI Threshold")) -> ()  [unwired: 2 in, 2 out]
          }
          event "Toggle\nMeasurement": Value Change {
            n174 = event-data() -> ("NewVal"=w447:bool)  [unwired: 1 in, 5 out]
            n175 = flat-sequence {
              tunnel: [w458] -> w446
              tunnel: w447 -> [w468]
              tunnel: w446 -> [w466]
              frame #0 {
                n176 = local read "Measurement\nActive"() -> (w459:bool)
                n177 = local write "Hardware\nBusy"(TRUE ("Hardware\nBusy")) -> ()
                n178 = Wait (ms)(milliseconds to wait=u32 3000) -> ()  [unwired: 1 out]
                n179 = local read "FlexCompute\nDevices"() -> (w457:string[][])
                n180 = local read "FlexSDR\nDevices"() -> (w455:string[][])
                n181 = Not(x=w459) -> (.not. x?=w458:bool)
                n182 = local read "RTHost\nDevices"() -> (w456:string[][])
                n183 = property on="RTHost Selection" class="Ring (strict)"() -> ("Value"=w454:u16)  [unwired: 2 in, 2 out]
                n184 = property on="FlexSDR Selection" class="Ring (strict)"() -> ("Value"=w453:u16)  [unwired: 2 in, 2 out]
                n185 = property on="FlexCompute Selection" class="Ring (strict)"() -> ("Value"=w452:u16)  [unwired: 2 in, 2 out]
                n186 = Bundle By Name(cluster=T3 {"RTHost Selection"=0, "FlexCompute Selection"=0, "FlexSDR Selection"=0} ("Device Selection"), "RTHost Selection"=w454, "FlexCompute Selection"=w453, "FlexSDR Selection"=w452) -> (w449:T3)
                n187 = Bundle By Name(cluster=T4 {"RTHost\nDevices"=[["192.168.1.2", "FlexCompute C011T", "D83198"], ["192.168.1.4", "FlexCompute C011T", "50E219"]], "FlexCompute\nDevices"=[["192.168.1.1", "FlexCompute C100T", "909B13"], ["192.168.1.3", "FlexCompute C100T", "4363DA"]], "FlexSDR\nDevices"=[["192.168.1.5", "FlexSDR S8010-01", "9770BC"], ["192.168.1.6", "FlexSDR S8010-01", "24BD53"]]} ("Devices"), "RTHost\nDevices"=w456, "FlexCompute\nDevices"=w457, "FlexSDR\nDevices"=w455) -> (w448:T4)
                n188 = case shown="True" w458 {
                  tunnel: w449 -> [w462 w465]
                  tunnel: w448 -> [w463 w464]
                  frame True {
                    n189 = call "Device_Measurement_Start.vi"("Device Selection"=w462, "Devices"=w463) -> ()  [unwired: 2 in]
                  }
                  frame False {
                    n190 = call "Device_Measurement_Stop.vi"("Device Selection"=w465, "Devices"=w464) -> ()  [unwired: 2 in]
                  }
                }
              }
              frame #1 {
                n191 = Not(x=w468) -> (.not. x?=w467:bool)
                n192 = local write "Hardware\nBusy"(FALSE ("Hardware\nBusy")) -> ()
                n193 = local write "Toggle\nMeasurement"(w467) -> ()
                n194 = local write "Measurement\nActive"(w466) -> ()
              }
            }
          }
        }
        n195 = local read "Stop Program"() -> (w170:bool)
      }
      n196 = while {
        stop <- w9 stop-if-true
        n197 = local read "Measurement\nActive"() -> (w8:bool)
        n198 = local read "WRx 1 En"() -> (w7:bool)
        n199 = local read "WRx 2 En"() -> (w6:bool)
        n200 = case shown="True" w8 {
          tunnel: w7 -> [_ w11]
          tunnel: w6 -> [_ w10]
          frame False {
          }
          frame True {
            n201 = flat-sequence {
              tunnel: w11 -> [w13]
              tunnel: w10 -> [w15]
              frame #0 {
                n202 = case shown="False" w13 {
                  tunnel: [w16 w57] -> w12
                  frame False {
                    n203 = property on="WRx 1 Spectrum Plot" class="XYGraph (strict)"() -> ("XScale.Maximum"=w20:dbl)  [unwired: 2 in, 2 out]
                    n204 = Divide(x=w20, y=10000000.0) -> (x/y=w18:dbl)
                    n205 = case shown="365, 400" w18 {
                      tunnel: [w22 w33 w44] -> w16
                      tunnel: dbl[] [-80.0, -80.0, -80.0, -80.0, -80.0, -80.0, -80.0, -80.0, -80.0, -80.0, -80.0, -80.0, -80.0, -80.0, -80.0, -80.0, -80.0, -80.0, -80.0, -80.0, -80.0, -80.0, -80.0, -80.0, -80.0, -80.0, -80.0, -80.0, -80.0, -80.0, -80.0, -80.0, -80.0, -80.0, -80.0, -80.0, -80.0, -80.0, -80.0, -80.0, -80.0, -80.0, -80.0, -80.0, -80.0, -80.0, -80.0, -80.0, -80.0, -80.0, -80.0, -80.0, -80.0, -80.0, -80.0, -80.0, -80.0, -80.0, -80.0, -80.0, -80.0, -80.0, -80.0, -80.0, -80.0, -80.0, -80.0, -80.0, -80.0, -80.0, -80.0, -80.0, -80.0, -80.0, -80.0, -80.0, -80.0, -80.0, -80.0, -80.0, -80.0] ("Array 3") -> [w21 w32 w43]
                      frame 160, Default {
                        w25 = 81 ("samples")
                        n206 = call-poly <vilib>:"Ramp Pattern.vi"("start"=800000000.0, "end"=1600000000.0, "samples"=w25) -> ("Ramp Pattern"=w29:dbl[])  [unwired: 7 in, 1 out]
                        n207 = call <vilib>:"Uniform White Noise.vi"("amplitude"=0.0, "samples"=w25) -> ("uniform white noise"=w24:dbl[])  [unwired: 8 in, 1 out]
                        n208 = call "Convert to Dynamic Data"("Array"=w29) -> ("Dynamic Data Type"=w30:dynamicdata)  [unwired: 3 in]
                        n209 = Add(x=w24, y=w21) -> (x+y=w23:dbl[])
                        n210 = call "Convert to Dynamic Data2"("Array"=w23) -> ("Dynamic Data Type"=w31:dynamicdata)  [unwired: 3 in]
                        n211 = call "Build XY Graph"("Y Input"=w31, "X Input"=w30) -> ("XY Graph"=w22:cluster{"X":dbl[], "Y":dbl[]}[])  [unwired: 8 in, 1 out]
                      }
                      frame 180 {
                        w36 = 81 ("samples")
                        n212 = call-poly <vilib>:"Ramp Pattern.vi"("start"=1000000000.0, "end"=1800000000.0, "samples"=w36) -> ("Ramp Pattern"=w40:dbl[])  [unwired: 7 in, 1 out]
                        n213 = call <vilib>:"Uniform White Noise.vi"("amplitude"=0.0, "samples"=w36) -> ("uniform white noise"=w35:dbl[])  [unwired: 8 in, 1 out]
                        n214 = call "Convert to Dynamic Data15"("Array"=w40) -> ("Dynamic Data Type"=w41:dynamicdata)  [unwired: 3 in]
                        n215 = Add(x=w35, y=w32) -> (x+y=w34:dbl[])
                        n216 = call "Convert to Dynamic Data16"("Array"=w34) -> ("Dynamic Data Type"=w42:dynamicdata)  [unwired: 3 in]
                        n217 = call "Build XY Graph8"("Y Input"=w42, "X Input"=w41) -> ("XY Graph"=w33:cluster{"X":dbl[], "Y":dbl[]}[])  [unwired: 8 in, 1 out]
                      }
                      frame 365, 400 {
                        w47 = 81 ("samples")
                        n218 = call-poly <vilib>:"Ramp Pattern.vi"("start"=2350000000.0, "end"=3650000000.0, "samples"=w47) -> ("Ramp Pattern"=w51:dbl[])  [unwired: 7 in, 1 out]
                        n219 = call <vilib>:"Uniform White Noise.vi"("amplitude"=0.0, "samples"=w47) -> ("uniform white noise"=w46:dbl[])  [unwired: 8 in, 1 out]
                        n220 = call "Convert to Dynamic Data17"("Array"=w51) -> ("Dynamic Data Type"=w52:dynamicdata)  [unwired: 3 in]
                        n221 = Add(x=w46, y=w43) -> (x+y=w45:dbl[])
                        n222 = call "Convert to Dynamic Data18"("Array"=w45) -> ("Dynamic Data Type"=w53:dynamicdata)  [unwired: 3 in]
                        n223 = call "Build XY Graph9"("Y Input"=w53, "X Input"=w52) -> ("XY Graph"=w44:cluster{"X":dbl[], "Y":dbl[]}[])  [unwired: 8 in, 1 out]
                      }
                    }
                  }
                  frame True {
                    n224 = property on="WRx 1 Spectrum Plot" class="XYGraph (strict)"() -> ("XScale.Maximum"=w56:dbl)  [unwired: 2 in, 2 out]
                    n225 = Divide(x=w56, y=10000000.0) -> (x/y=w54:dbl)
                    n226 = case shown="365, 400" w54 {
                      tunnel: [w58 w69 w81] -> w57
                      frame 160, Default {
                        w62 = 81 ("samples")
                        n227 = call-poly <vilib>:"Ramp Pattern.vi"("start"=800000000.0, "end"=1600000000.0, "samples"=w62) -> ("Ramp Pattern"=w66:dbl[])  [unwired: 7 in, 1 out]
                        n228 = call <vilib>:"Uniform White Noise.vi"("amplitude"=1.0, "samples"=w62) -> ("uniform white noise"=w61:dbl[])  [unwired: 8 in, 1 out]
                        n229 = call "Convert to Dynamic Data19"("Array"=w66) -> ("Dynamic Data Type"=w67:dynamicdata)  [unwired: 3 in]
                        n230 = Add(x=w61, y=dbl[] [-80.0, -80.0, -80.0, -80.0, -80.0, -80.0, -80.0, -80.0, -80.0, -80.0, -80.0, -80.0, -80.0, -80.0, -80.0, -40.0, -40.0, -40.0, -40.0, -40.0, -40.0, -40.0, -40.0, -40.0, -40.0, -40.0, -40.0, -40.0, -40.0, -40.0, -40.0, -40.0, -40.0, -40.0, -40.0, -40.0, -40.0, -40.0, -40.0, -40.0, -40.0, -40.0, -40.0, -40.0, -40.0, -40.0, -40.0, -40.0, -40.0, -40.0, -40.0, -40.0, -40.0, -40.0, -40.0, -40.0, -40.0, -40.0, -40.0, -40.0, -40.0, -40.0, -40.0, -40.0, -40.0, -40.0, -80.0, -80.0, -80.0, -80.0, -80.0, -80.0, -80.0, -80.0, -80.0, -80.0, -80.0, -80.0, -80.0, -80.0, -80.0] ("Array")) -> (x+y=w59:dbl[])
                        n231 = call "Convert to Dynamic Data20"("Array"=w59) -> ("Dynamic Data Type"=w68:dynamicdata)  [unwired: 3 in]
                        n232 = call "Build XY Graph10"("Y Input"=w68, "X Input"=w67) -> ("XY Graph"=w58:cluster{"X":dbl[], "Y":dbl[]}[])  [unwired: 8 in, 1 out]
                      }
                      frame 180 {
                        w73 = 81 ("samples")
                        n233 = call-poly <vilib>:"Ramp Pattern.vi"("start"=1000000000.0, "end"=1800000000.0, "samples"=w73) -> ("Ramp Pattern"=w77:dbl[])  [unwired: 7 in, 1 out]
                        n234 = call <vilib>:"Uniform White Noise.vi"("amplitude"=1.0, "samples"=w73) -> ("uniform white noise"=w72:dbl[])  [unwired: 8 in, 1 out]
                        n235 = call "Convert to Dynamic Data21"("Array"=w77) -> ("Dynamic Data Type"=w78:dynamicdata)  [unwired: 3 in]
                        n236 = Add(x=w72, y=dbl[] [-80.0, -80.0, -80.0, -80.0, -80.0, -80.0, -80.0, -80.0, -80.0, -80.0, -80.0, -80.0, -80.0, -80.0, -80.0, -40.0, -40.0, -40.0, -40.0, -40.0, -40.0, -40.0, -40.0, -40.0, -40.0, -40.0, -40.0, -40.0, -40.0, -40.0, -40.0, -40.0, -40.0, -40.0, -40.0, -40.0, -40.0, -40.0, -40.0, -40.0, -40.0, -40.0, -40.0, -40.0, -40.0, -40.0, -40.0, -40.0, -40.0, -40.0, -40.0, -40.0, -40.0, -40.0, -40.0, -40.0, -40.0, -40.0, -40.0, -40.0, -40.0, -40.0, -40.0, -40.0, -40.0, -40.0, -80.0, -80.0, -80.0, -80.0, -80.0, -80.0, -80.0, -80.0, -80.0, -80.0, -80.0, -80.0, -80.0, -80.0, -80.0] ("Array")) -> (x+y=w70:dbl[])
                        n237 = call "Convert to Dynamic Data22"("Array"=w70) -> ("Dynamic Data Type"=w79:dynamicdata)  [unwired: 3 in]
                        n238 = call "Build XY Graph11"("Y Input"=w79, "X Input"=w78) -> ("XY Graph"=w69:cluster{"X":dbl[], "Y":dbl[]}[])  [unwired: 8 in, 1 out]
                      }
                      frame 365, 400 {
                        w84 = 81 ("samples")
                        n239 = call-poly <vilib>:"Ramp Pattern.vi"("start"=2350000000.0, "end"=3650000000.0, "samples"=w84) -> ("Ramp Pattern"=w88:dbl[])  [unwired: 7 in, 1 out]
                        n240 = call <vilib>:"Uniform White Noise.vi"("amplitude"=1.0, "samples"=w84) -> ("uniform white noise"=w83:dbl[])  [unwired: 8 in, 1 out]
                        n241 = call "Convert to Dynamic Data23"("Array"=w88) -> ("Dynamic Data Type"=w89:dynamicdata)  [unwired: 3 in]
                        n242 = Add(x=w83, y=dbl[] [-80.0, -80.0, -80.0, -80.0, -80.0, -80.0, -80.0, -80.0, -80.0, -80.0, -40.0, -40.0, -40.0, -40.0, -40.0, -40.0, -40.0, -40.0, -40.0, -40.0, -40.0, -40.0, -40.0, -40.0, -40.0, -40.0, -40.0, -40.0, -40.0, -40.0, -40.0, -40.0, -40.0, -40.0, -40.0, -40.0, -40.0, -40.0, -40.0, -40.0, -40.0, -40.0, -40.0, -40.0, -40.0, -40.0, -40.0, -40.0, -40.0, -40.0, -40.0, -40.0, -40.0, -40.0, -40.0, -40.0, -40.0, -40.0, -40.0, -40.0, -40.0, -40.0, -40.0, -40.0, -40.0, -40.0, -40.0, -40.0, -40.0, -40.0, -40.0, -80.0, -80.0, -80.0, -80.0, -80.0, -80.0, -80.0, -80.0, -80.0, -80.0] ("Array 2")) -> (x+y=w82:dbl[])
                        n243 = call "Convert to Dynamic Data24"("Array"=w82) -> ("Dynamic Data Type"=w90:dynamicdata)  [unwired: 3 in]
                        n244 = call "Build XY Graph12"("Y Input"=w90, "X Input"=w89) -> ("XY Graph"=w81:cluster{"X":dbl[], "Y":dbl[]}[])  [unwired: 8 in, 1 out]
                      }
                    }
                  }
                }
                n245 = case shown="False" w15 {
                  tunnel: [w91 w132] -> w14
                  frame False {
                    n246 = property on="WRx 2 Spectrum Plot" class="XYGraph (strict)"() -> ("XScale.Maximum"=w95:dbl)  [unwired: 2 in, 2 out]
                    n247 = Divide(x=w95, y=10000000.0) -> (x/y=w93:dbl)
                    n248 = case shown="365, 400" w93 {
                      tunnel: [w97 w108 w119] -> w91
                      tunnel: dbl[] [-80.0, -80.0, -80.0, -80.0, -80.0, -80.0, -80.0, -80.0, -80.0, -80.0, -80.0, -80.0, -80.0, -80.0, -80.0, -80.0, -80.0, -80.0, -80.0, -80.0, -80.0, -80.0, -80.0, -80.0, -80.0, -80.0, -80.0, -80.0, -80.0, -80.0, -80.0, -80.0, -80.0, -80.0, -80.0, -80.0, -80.0, -80.0, -80.0, -80.0, -80.0, -80.0, -80.0, -80.0, -80.0, -80.0, -80.0, -80.0, -80.0, -80.0, -80.0, -80.0, -80.0, -80.0, -80.0, -80.0, -80.0, -80.0, -80.0, -80.0, -80.0, -80.0, -80.0, -80.0, -80.0, -80.0, -80.0, -80.0, -80.0, -80.0, -80.0, -80.0, -80.0, -80.0, -80.0, -80.0, -80.0, -80.0, -80.0, -80.0, -80.0] ("Array 3") -> [w96 w107 w118]
                      frame 160, Default {
                        w100 = 81 ("samples")
                        n249 = call-poly <vilib>:"Ramp Pattern.vi"("start"=800000000.0, "end"=1600000000.0, "samples"=w100) -> ("Ramp Pattern"=w104:dbl[])  [unwired: 7 in, 1 out]
                        n250 = call <vilib>:"Uniform White Noise.vi"("amplitude"=0.0, "samples"=w100) -> ("uniform white noise"=w99:dbl[])  [unwired: 8 in, 1 out]
                        n251 = call "Convert to Dynamic Data9"("Array"=w104) -> ("Dynamic Data Type"=w105:dynamicdata)  [unwired: 3 in]
                        n252 = Add(x=w99, y=w96) -> (x+y=w98:dbl[])
                        n253 = call "Convert to Dynamic Data10"("Array"=w98) -> ("Dynamic Data Type"=w106:dynamicdata)  [unwired: 3 in]
                        n254 = call "Build XY Graph5"("Y Input"=w106, "X Input"=w105) -> ("XY Graph"=w97:cluster{"X":dbl[], "Y":dbl[]}[])  [unwired: 8 in, 1 out]
                      }
                      frame 180 {
                        w111 = 81 ("samples")
                        n255 = call-poly <vilib>:"Ramp Pattern.vi"("start"=1000000000.0, "end"=1800000000.0, "samples"=w111) -> ("Ramp Pattern"=w115:dbl[])  [unwired: 7 in, 1 out]
                        n256 = call <vilib>:"Uniform White Noise.vi"("amplitude"=0.0, "samples"=w111) -> ("uniform white noise"=w110:dbl[])  [unwired: 8 in, 1 out]
                        n257 = call "Convert to Dynamic Data11"("Array"=w115) -> ("Dynamic Data Type"=w116:dynamicdata)  [unwired: 3 in]
                        n258 = Add(x=w110, y=w107) -> (x+y=w109:dbl[])
                        n259 = call "Convert to Dynamic Data12"("Array"=w109) -> ("Dynamic Data Type"=w117:dynamicdata)  [unwired: 3 in]
                        n260 = call "Build XY Graph6"("Y Input"=w117, "X Input"=w116) -> ("XY Graph"=w108:cluster{"X":dbl[], "Y":dbl[]}[])  [unwired: 8 in, 1 out]
                      }
                      frame 365, 400 {
                        w122 = 81 ("samples")
                        n261 = call-poly <vilib>:"Ramp Pattern.vi"("start"=2350000000.0, "end"=3650000000.0, "samples"=w122) -> ("Ramp Pattern"=w126:dbl[])  [unwired: 7 in, 1 out]
                        n262 = call <vilib>:"Uniform White Noise.vi"("amplitude"=0.0, "samples"=w122) -> ("uniform white noise"=w121:dbl[])  [unwired: 8 in, 1 out]
                        n263 = call "Convert to Dynamic Data13"("Array"=w126) -> ("Dynamic Data Type"=w127:dynamicdata)  [unwired: 3 in]
                        n264 = Add(x=w121, y=w118) -> (x+y=w120:dbl[])
                        n265 = call "Convert to Dynamic Data14"("Array"=w120) -> ("Dynamic Data Type"=w128:dynamicdata)  [unwired: 3 in]
                        n266 = call "Build XY Graph7"("Y Input"=w128, "X Input"=w127) -> ("XY Graph"=w119:cluster{"X":dbl[], "Y":dbl[]}[])  [unwired: 8 in, 1 out]
                      }
                    }
                  }
                  frame True {
                    n267 = property on="WRx 2 Spectrum Plot" class="XYGraph (strict)"() -> ("XScale.Maximum"=w131:dbl)  [unwired: 2 in, 2 out]
                    n268 = Divide(x=w131, y=10000000.0) -> (x/y=w129:dbl)
                    n269 = case shown="365, 400" w129 {
                      tunnel: [w133 w144 w156] -> w132
                      frame 160, Default {
                        w137 = 81 ("samples")
                        n270 = call-poly <vilib>:"Ramp Pattern.vi"("start"=800000000.0, "end"=1600000000.0, "samples"=w137) -> ("Ramp Pattern"=w141:dbl[])  [unwired: 7 in, 1 out]
                        n271 = call <vilib>:"Uniform White Noise.vi"("amplitude"=1.0, "samples"=w137) -> ("uniform white noise"=w136:dbl[])  [unwired: 8 in, 1 out]
                        n272 = call "Convert to Dynamic Data3"("Array"=w141) -> ("Dynamic Data Type"=w142:dynamicdata)  [unwired: 3 in]
                        n273 = Add(x=w136, y=dbl[] [-80.0, -80.0, -80.0, -80.0, -80.0, -80.0, -80.0, -80.0, -80.0, -80.0, -80.0, -80.0, -80.0, -80.0, -80.0, -40.0, -40.0, -40.0, -40.0, -40.0, -40.0, -40.0, -40.0, -40.0, -40.0, -40.0, -40.0, -40.0, -40.0, -40.0, -40.0, -40.0, -40.0, -40.0, -40.0, -40.0, -40.0, -40.0, -40.0, -40.0, -40.0, -40.0, -40.0, -40.0, -40.0, -40.0, -40.0, -40.0, -40.0, -40.0, -40.0, -40.0, -40.0, -40.0, -40.0, -40.0, -40.0, -40.0, -40.0, -40.0, -40.0, -40.0, -40.0, -40.0, -40.0, -40.0, -80.0, -80.0, -80.0, -80.0, -80.0, -80.0, -80.0, -80.0, -80.0, -80.0, -80.0, -80.0, -80.0, -80.0, -80.0] ("Array")) -> (x+y=w134:dbl[])
                        n274 = call "Convert to Dynamic Data4"("Array"=w134) -> ("Dynamic Data Type"=w143:dynamicdata)  [unwired: 3 in]
                        n275 = call "Build XY Graph2"("Y Input"=w143, "X Input"=w142) -> ("XY Graph"=w133:cluster{"X":dbl[], "Y":dbl[]}[])  [unwired: 8 in, 1 out]
                      }
                      frame 180 {
                        w148 = 81 ("samples")
                        n276 = call-poly <vilib>:"Ramp Pattern.vi"("start"=1000000000.0, "end"=1800000000.0, "samples"=w148) -> ("Ramp Pattern"=w152:dbl[])  [unwired: 7 in, 1 out]
                        n277 = call <vilib>:"Uniform White Noise.vi"("amplitude"=1.0, "samples"=w148) -> ("uniform white noise"=w147:dbl[])  [unwired: 8 in, 1 out]
                        n278 = call "Convert to Dynamic Data5"("Array"=w152) -> ("Dynamic Data Type"=w153:dynamicdata)  [unwired: 3 in]
                        n279 = Add(x=w147, y=dbl[] [-80.0, -80.0, -80.0, -80.0, -80.0, -80.0, -80.0, -80.0, -80.0, -80.0, -80.0, -80.0, -80.0, -80.0, -80.0, -40.0, -40.0, -40.0, -40.0, -40.0, -40.0, -40.0, -40.0, -40.0, -40.0, -40.0, -40.0, -40.0, -40.0, -40.0, -40.0, -40.0, -40.0, -40.0, -40.0, -40.0, -40.0, -40.0, -40.0, -40.0, -40.0, -40.0, -40.0, -40.0, -40.0, -40.0, -40.0, -40.0, -40.0, -40.0, -40.0, -40.0, -40.0, -40.0, -40.0, -40.0, -40.0, -40.0, -40.0, -40.0, -40.0, -40.0, -40.0, -40.0, -40.0, -40.0, -80.0, -80.0, -80.0, -80.0, -80.0, -80.0, -80.0, -80.0, -80.0, -80.0, -80.0, -80.0, -80.0, -80.0, -80.0] ("Array")) -> (x+y=w145:dbl[])
                        n280 = call "Convert to Dynamic Data6"("Array"=w145) -> ("Dynamic Data Type"=w154:dynamicdata)  [unwired: 3 in]
                        n281 = call "Build XY Graph3"("Y Input"=w154, "X Input"=w153) -> ("XY Graph"=w144:cluster{"X":dbl[], "Y":dbl[]}[])  [unwired: 8 in, 1 out]
                      }
                      frame 365, 400 {
                        w159 = 81 ("samples")
                        n282 = call-poly <vilib>:"Ramp Pattern.vi"("start"=2350000000.0, "end"=3650000000.0, "samples"=w159) -> ("Ramp Pattern"=w163:dbl[])  [unwired: 7 in, 1 out]
                        n283 = call <vilib>:"Uniform White Noise.vi"("amplitude"=1.0, "samples"=w159) -> ("uniform white noise"=w158:dbl[])  [unwired: 8 in, 1 out]
                        n284 = call "Convert to Dynamic Data7"("Array"=w163) -> ("Dynamic Data Type"=w164:dynamicdata)  [unwired: 3 in]
                        n285 = Add(x=w158, y=dbl[] [-80.0, -80.0, -80.0, -80.0, -80.0, -80.0, -80.0, -80.0, -80.0, -80.0, -40.0, -40.0, -40.0, -40.0, -40.0, -40.0, -40.0, -40.0, -40.0, -40.0, -40.0, -40.0, -40.0, -40.0, -40.0, -40.0, -40.0, -40.0, -40.0, -40.0, -40.0, -40.0, -40.0, -40.0, -40.0, -40.0, -40.0, -40.0, -40.0, -40.0, -40.0, -40.0, -40.0, -40.0, -40.0, -40.0, -40.0, -40.0, -40.0, -40.0, -40.0, -40.0, -40.0, -40.0, -40.0, -40.0, -40.0, -40.0, -40.0, -40.0, -40.0, -40.0, -40.0, -40.0, -40.0, -40.0, -40.0, -40.0, -40.0, -40.0, -40.0, -80.0, -80.0, -80.0, -80.0, -80.0, -80.0, -80.0, -80.0, -80.0, -80.0] ("Array 2")) -> (x+y=w157:dbl[])
                        n286 = call "Convert to Dynamic Data8"("Array"=w157) -> ("Dynamic Data Type"=w165:dynamicdata)  [unwired: 3 in]
                        n287 = call "Build XY Graph4"("Y Input"=w165, "X Input"=w164) -> ("XY Graph"=w156:cluster{"X":dbl[], "Y":dbl[]}[])  [unwired: 8 in, 1 out]
                      }
                    }
                  }
                }
                n288 = local write "WRx 1 Spectrum Plot"(w12) -> ()
                n289 = local write "WRx 2 Spectrum Plot"(w14) -> ()
              }
              frame #1 {
                n290 = local read "Spectrum Sampling Period (s)"() -> (w166:dbl)
                n291 = Multiply(x=w166, y=1000.0) -> (x*y=w168:dbl)
                n292 = Wait (ms)(milliseconds to wait=w168) -> ()  [unwired: 1 out]
              }
            }
          }
        }
        n293 = local read "Stop Program"() -> (w9:bool)
      }
    }
    frame #1 {
      n294 = Wait (ms)(milliseconds to wait=u32 1000) -> ()  [unwired: 1 out]
    }
    frame #2 {
      w471 = FALSE ("Stop Program")
      # "Procedure\nTo Properly\nDisconnect"
      n295 = local write "Stop Program"(w471) -> ()
      n296 = local write "Measurement\nActive"(w471) -> ()
    }
  }
  n297 = flat-sequence {
    tunnel: [w473] -> w4
    tunnel: [w481] -> w5
    tunnel: w4 -> [w481]
    tunnel: [w480] -> w1
    tunnel: w5 -> [w489]
    tunnel: [w489] -> w3
    tunnel: w1 -> [w488]
    tunnel: w3 -> [w496]
    tunnel: [w496] -> w2
    tunnel: w2 -> [w502]
    frame #0 {
      w474 = FALSE ("Scan for\nConfig")
      w475 = FALSE ("GPS \nLOCK")
      w479 = u16 0 items=[""] ("RTHost Selection")
      w477 = string[][] [] ("Flex Computer\nDevices 2")
      w478 = string[] [] ("Strings []")
      w473 = T2."Disabled and Grayed Out" ("Disabled")
      n298 = property on="FlexSDR Selection" class="Ring (strict)"("Strings []"=w478, "Value"=w479) -> ()  [unwired: 2 in, 2 out]
      n299 = property on="FlexCompute Selection" class="Ring (strict)"("Strings []"=w478, "Value"=w479) -> ()  [unwired: 2 in, 2 out]
      n300 = property on="RTHost Selection" class="Ring (strict)"("Strings []"=w478, "Value"=w479) -> ()  [unwired: 2 in, 2 out]
      n301 = local write "RTHost\nDevices"(w477) -> ()
      n302 = local write "FlexCompute\nDevices"(w477) -> ()
      n303 = local write "Hardware\nBusy"(w475) -> ()
      n304 = local write "FlexSDR\nDevices"(w477) -> ()
      n305 = local write "GPS \nLOCK"(w475) -> ()
      n306 = local write "Spectrum Sampling Period (s)"(0.25 ("Spectrum Sampling Period (s)")) -> ()
      n307 = local write "Measurement\nActive"(FALSE ("Measurement\nActive")) -> ()
      n308 = property on="Scan for\nConfig" class="Bool (strict)"("DisabledEnum"=w473, "Value"=w474) -> ()  [unwired: 2 in, 2 out]
      n309 = property on="Toggle\nMeasurement" class="Bool (strict)"("DisabledEnum"=w473, "Value"=w474) -> ()  [unwired: 2 in, 2 out]
    }
    frame #1 {
      w480 = string[] ["500 MHz"] ("Strings []")
      w486 = u16 0 items=["500 MHz"] ("WRx 1\nBandwidth Mode")
      w485 = u16 0 items=["Automatic", "Fixed"] ("OBRx 1\nGain Mode")
      w487 = u16 0 items=["1200 MHz", "1400 MHz", "3000 MHZ"] ("OBRx 1\nIF Frequency")
      n310 = property on="WRx 1\nEnable Channel" class="Bool (strict)"("DisabledEnum"=w481, "Value"=FALSE ("OBRx 1\nEnable Channel")) -> ()  [unwired: 2 in, 2 out]
      n311 = property on="WRx 1\nIF Frequency" class="Ring (strict)"("DisabledEnum"=w481, "Value"=w487) -> ()  [unwired: 2 in, 2 out]
      n312 = property on="WRx 1\nBandwidth Mode" class="Ring (strict)"("DisabledEnum"=w481, "Value"=w486, "Strings []"=w480) -> ()  [unwired: 2 in, 2 out]
      n313 = property on="WRx 1\nGain Mode" class="Ring (strict)"("DisabledEnum"=w481, "Value"=w485) -> ()  [unwired: 2 in, 2 out]
      n314 = property on="WRx 1\nGain Attenuation" class="Knob (strict)"("DisabledEnum"=w481, "Value"=i64 0 ("WRx 1\nGain Attenuation")) -> ()  [unwired: 2 in, 2 out]
      n315 = property on="WRx 1\nRSSI Threshold" class="DigNum (strict)"("DisabledEnum"=w481, "Value"=-20.0 ("WRx 1\nRSSI Threshold")) -> ()  [unwired: 2 in, 2 out]
    }
    frame #2 {
      w494 = u16 0 items=["500 MHz"] ("WRx 1\nBandwidth Mode")
      w493 = u16 0 items=["Automatic", "Fixed"] ("OBRx 1\nGain Mode")
      w495 = u16 0 items=["1200 MHz", "1400 MHz", "3000 MHZ"] ("OBRx 1\nIF Frequency")
      n316 = property on="WRx 2\nIF Frequency" class="Ring (strict)"("DisabledEnum"=w489, "Value"=w495) -> ()  [unwired: 2 in, 2 out]
      n317 = property on="WRx 2\nBandwidth Mode" class="Ring (strict)"("DisabledEnum"=w489, "Value"=w494, "Strings []"=w488) -> ()  [unwired: 2 in, 2 out]
      n318 = property on="WRx 2\nGain Mode" class="Ring (strict)"("DisabledEnum"=w489, "Value"=w493) -> ()  [unwired: 2 in, 2 out]
      n319 = property on="WRx 2\nGain Attenuation" class="Knob (strict)"("DisabledEnum"=w489, "Value"=i64 0 ("WRx 1\nGain Attenuation")) -> ()  [unwired: 2 in, 2 out]
      n320 = property on="WRx 2\nRSSI Threshold" class="DigNum (strict)"("DisabledEnum"=w489, "Value"=-20.0 ("WRx 1\nRSSI Threshold")) -> ()  [unwired: 2 in, 2 out]
      n321 = property on="WRx 2\nEnable Channel" class="Bool (strict)"("DisabledEnum"=w489, "Value"=FALSE ("OBRx 1\nEnable Channel")) -> ()  [unwired: 2 in, 2 out]
    }
    frame #3 {
      w497 = FALSE ("Runtime\nCalibration")
      w500 = u16 0 items=["Single", "Continuous"] ("Trigger Frequency")
      w501 = u16 0 items=["GPS Time", "Anamoly Detection"] ("Trigger Type")
      n322 = property on="Runtime\nCalibration" class="Bool (strict)"("DisabledEnum"=w496, "Value"=w497) -> ()  [unwired: 2 in, 2 out]
      n323 = property on="Doppler\nBypass" class="Bool (strict)"("DisabledEnum"=w496, "Value"=w497) -> ()  [unwired: 2 in, 2 out]
      n324 = property on="Trigger Type" class="Ring (strict)"("DisabledEnum"=w496, "Value"=w501) -> ()  [unwired: 2 in, 2 out]
      n325 = property on="Trigger Frequency" class="Ring (strict)"("DisabledEnum"=w496, "Value"=w500) -> ()  [unwired: 2 in, 2 out]
      n326 = property on="Update \nConfiguration" class="Bool (strict)"("DisabledEnum"=w496, "Value"=w497) -> ()  [unwired: 2 in, 2 out]
      n327 = property on="Pre-Trigger Time" class="DigNum (strict)"("DisabledEnum"=w496, "Value"=0.25 ("Pre-Trigger Time")) -> ()  [unwired: 2 in, 2 out]
      n328 = property on="Post-Trigger Time" class="DigNum (strict)"("DisabledEnum"=w496, "Value"=1.0 ("Post-Trigger Time")) -> ()  [unwired: 2 in, 2 out]
    }
    frame #4 {
      w503 = 0.0 ("WRx 1 RSSI")
      w504 = FALSE ("HW Reset")
      n329 = property on="WRx 2 \nGain Attenuation" class="DigNum (strict)"("DisabledEnum"=w502, "Value"=w503) -> ()  [unwired: 2 in, 2 out]
      n330 = property on="Self-Cal" class="Bool (strict)"("DisabledEnum"=w502, "Value"=w504) -> ()  [unwired: 2 in, 2 out]
      n331 = property on="HW Reset" class="Bool (strict)"("DisabledEnum"=w502, "Value"=w504) -> ()  [unwired: 2 in, 2 out]
      n332 = property on="WRx Scan" class="Bool (strict)"("DisabledEnum"=w502, "Value"=w504) -> ()  [unwired: 2 in, 2 out]
      n333 = property on="WRx 1 RSSI" class="DigNum (strict)"("DisabledEnum"=w502, "Value"=w503) -> ()  [unwired: 2 in, 2 out]
      n334 = property on="WRx 2 RSSI" class="DigNum (strict)"("DisabledEnum"=w502, "Value"=w503) -> ()  [unwired: 2 in, 2 out]
      n335 = property on="WRx 1 \nGain Attenuation" class="DigNum (strict)"("DisabledEnum"=w502, "Value"=w503) -> ()  [unwired: 2 in, 2 out]
    }
  }
  n336 = flat-sequence {
    frame #0 {
      # "Controls\n&\nIndicators"
    }
  }
